vi "solar_voy_def Rename Packet.vi"(8 "error in (no error)":errorcluster, 9 "New Packet Names":string[](array[string]), 10 "Packet Names":string[](array[string]), 11 "Packets in":T1[](array[typedef]) {"last_time" format="%<%H:%M:%S%3u %m/%d/%y>T"}) -> (0 "error out":errorcluster, 3 "Packets out":T1[](array[typedef]) {"last_time" format="%<%H:%M:%S%3u %m/%d/%y>T"})   [LabVIEW 2018]
doc: "This renames the specified <b>Packet Names</b> with the <b>New Packet Names</b> if found."
uses:
  solar_voy_def_ctl ITEM TYPE.ctl
  type/solar_type Item Type.ctl
  solar_voy_def_ctl ITEM.ctl
  solar_voy_def_ctl PACKET_ID.ctl
  solar_voy_def_ctl PACKET.ctl
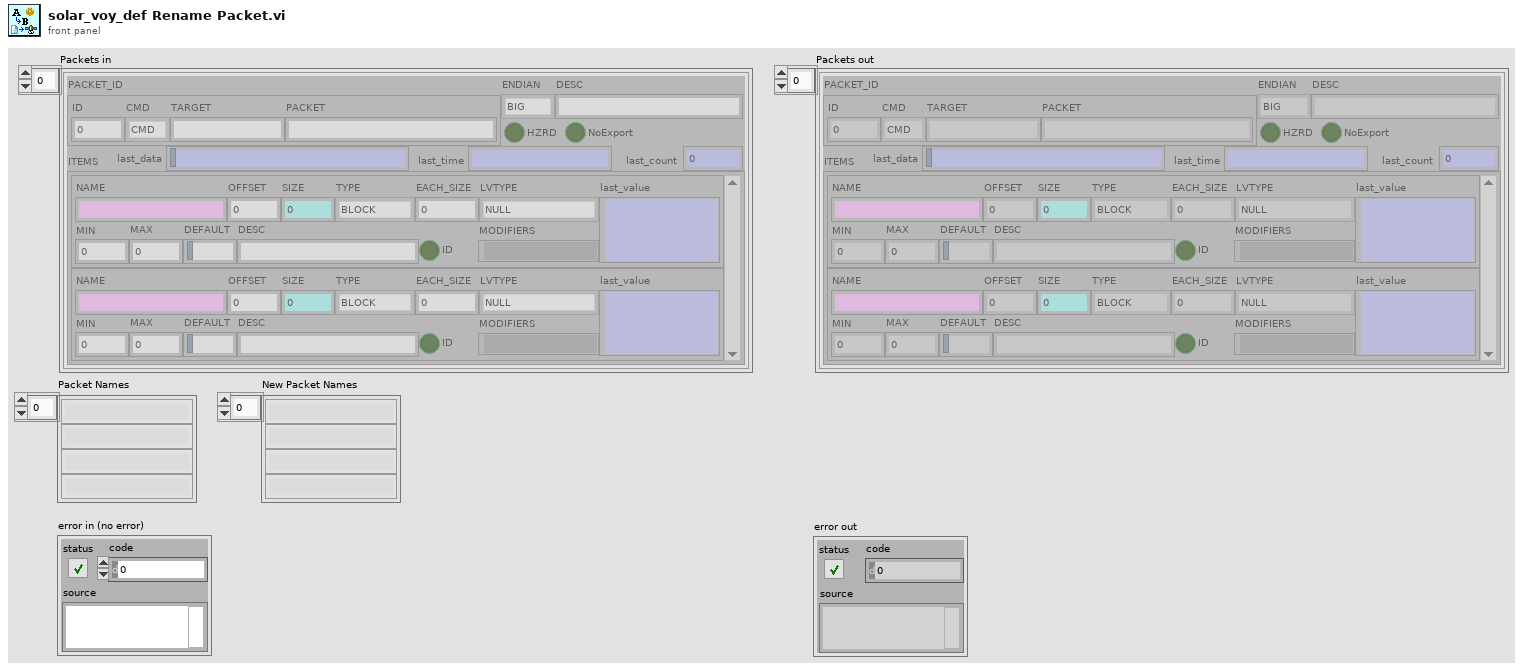
[diagram p1: front panel]
types:
  T1 = typedef "solar_voy_def_ctl PACKET.ctl" = cluster{"PACKET_ID":T2, "ENDIAN":enum8{"BIG", "LITTLE"}, "DESC":string, "HZRD":bool, "ITEMS":T3[], "NoExport":bool, "last_time":timestamp, "last_count":u32, "last_data":string}
  T2 = typedef "solar_voy_def_ctl PACKET_ID.ctl" = cluster{"ID":u16, "CMD":enum8{"CMD", "TLM"}, "TARGET":string, "PACKET":string}
  T3 = typedef "solar_voy_def_ctl ITEM.ctl" = cluster{"NAME":string, "OFFSET":i32, "SIZE":i32, "TYPE":T4, "EACH_SIZE":i32, "LVTYPE":T5, "MIN":dbl, "MAX":dbl, "DEFAULT":string, "DESC":string, "ID":bool, "MODIFIERS":variant, "last_value":variant}
  T4 = typedef "solar_voy_def_ctl ITEM TYPE.ctl" = enum8{"BLOCK", "INT", "UINT", "FLOAT", "STRING"}
  T5 = typedef "solar_type Item Type.ctl" = enum16{"NULL", "UNKNOWN", "CLUSTER", "I8", "I16", "I32", "I64", "U8", "U16", "U32", "U64", "U8_ENUM", "U16_ENUM", "U32_ENUM", "SGL", "DBL", "BOOLEAN", "STRING", "PATH", "VISA", "TAG", "TIME", "I8_1D", "I16_1D", "I32_1D", "I64_1D", "U8_1D", "U16_1D", "U32_1D", "U64_1D", "U8_ENUM_1D", "U16_ENUM_1D", "U32_ENUM_1D", "SGL_1D", "DBL_1D", "BOOLEAN_1D", "STRING_1D", "PATH_1D", "VISA_1D", "TAG_1D", "TIME_1D", "I8_2D", "I16_2D", "I32_2D", "I64_2D", "U8_2D", "U16_2D", "U32_2D", "U64_2D", "U8_ENUM_2D", "U16_ENUM_2D", "U32_ENUM_2D", "SGL_2D", "DBL_2D", "BOOLEAN_2D", "STRING_2D", "PATH_2D", "VISA_2D", "TAG_2D", "TIME_2D"}
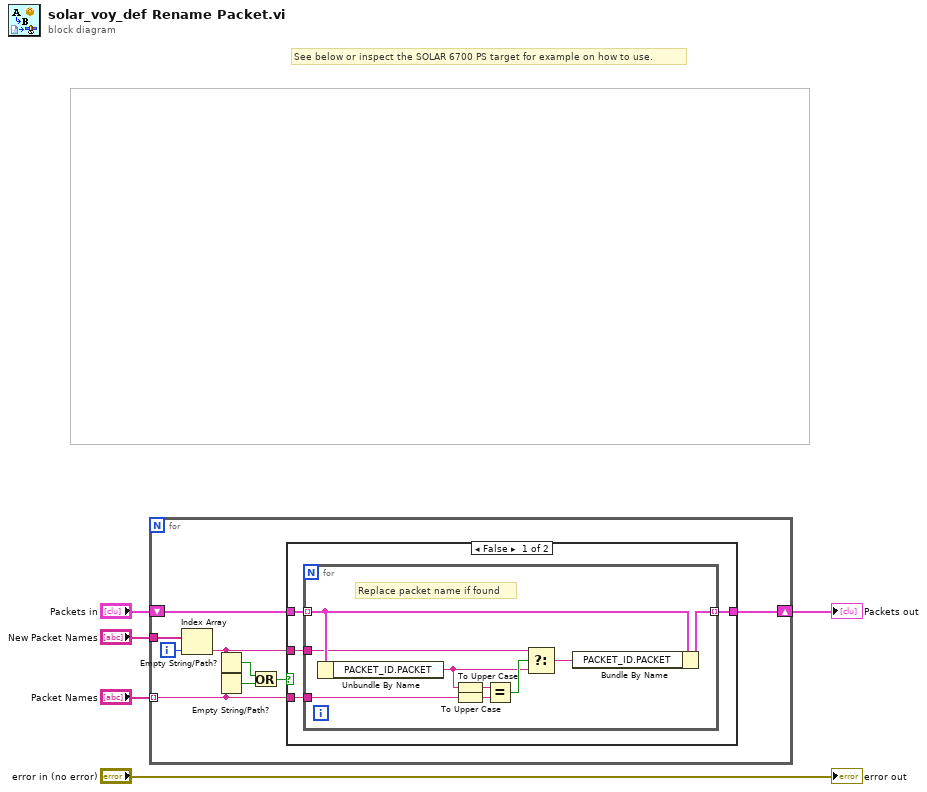
[diagram p0: block diagram]
diagram:
  # "See below or inspect the SOLAR 6700 PS target for example on how to use."
  n1 = for {
    tunnel: "Packet Names" -> [w12] mode=indexing
    tunnel: "New Packet Names" -> [w9]
    shift-right: [w13] -> w4
    shift-left: "Packets in" -> [w14]
    i -> [w6]
    n2 = Index Array(array=w9, index=w6) -> (element=w7:string)
    n3 = Empty String/Path?(string/path=w7) -> (empty?=w8:bool)
    n4 = Empty String/Path?(string/path=w12) -> (empty?=w11:bool)
    n5 = Or(x=w8, y=w11) -> (x .or. y?=w10:bool)
    n6 = case shown="False" w10 {
      tunnel: w14 -> [w18 w28]
      tunnel: [w17 w28] -> w13
      tunnel: w12 -> [w16 _]
      tunnel: w7 -> [w15 _]
      frame False {
        n7 = for {
          tunnel: w18 -> [w27] mode=indexing
          tunnel: [w26] -> w17 mode=indexing
          tunnel: w16 -> [w25]
          tunnel: w15 -> [w20]
          # "Replace packet name if found"
          n8 = Unbundle By Name(w27) -> ("PACKET_ID.PACKET"=w21:string)
          n9 = To Upper Case(1:w21) -> (0:w23:string)
          n10 = To Upper Case(1:w25) -> (0:w24:string)
          n11 = Equal?(x=w23, y=w24) -> (x = y?=w22:bool)
          n12 = Select(t=w20, s=w22, f=w21) -> (s? t:f=w19:string)
          n13 = Bundle By Name(cluster=w27, "PACKET_ID.PACKET"=w19) -> (w26:T1)
        }
      }
      frame True {
      }
    }
  }
  "Packets out" <- w4
  "error out" <- "error in (no error)"
